vi "Write Caller Notice Msg.vi"(8 "error in (no error)":errorcluster, 10 "Caller Notice Msg":refnum<class "Caller Notice Msg.lvclass">, 11 "Generic Actor in":refnum<class "Generic Actor.lvclass">) -> (0 "error out":errorcluster, 3 "Generic Actor out":refnum<class "Generic Actor.lvclass">)   [LabVIEW 2020, in "Generic Actor.lvlib" / "Generic Actor.lvclass"]
uses:
  Generic Actor.lvclass
  Generic Actor Messages/Caller Notice Msg/Caller Notice Msg.lvclass
  Generic Actor.lvclass/Generic Actor.ctl
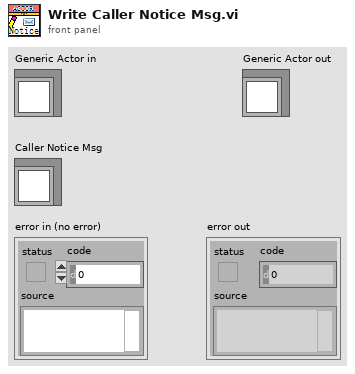
[diagram p1: front panel]
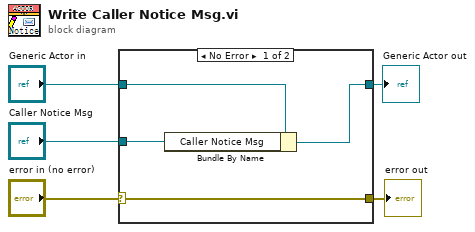
[diagram p0: block diagram]
diagram:
  n1 = case shown="No Error" "error in (no error)" {
    selector: "error in (no error)" -> [w6 w11]
    tunnel: "Generic Actor in" -> [w9 w10]
    tunnel: [w8 w10] -> w4
    tunnel: "Caller Notice Msg" -> [w7 _]
    tunnel: [w6 w11] -> w1
    frame No Error {
      n2 = Bundle By Name(cluster=w9, "Caller Notice Msg"=w7) -> (w8:refnum<class "Generic Actor.lvclass">)
    }
    frame Error {
    }
  }
  "Generic Actor out" <- w4
  "error out" <- w1
